vi "conditionalCheck.vi"(10 "State in":T1, 11 "CheckData in in":refnum<class "CheckData.lvclass">[](array[class])) -> (3 "CheckData out":refnum<class "CheckData.lvclass">[](array[class]))   [LabVIEW 2018, in "CheckData.lvclass"]
uses:
  CheckData.lvclass
  TypeDef_ControlState.ctl
  CheckData.lvclass/CheckData.ctl
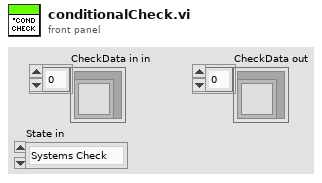
[diagram p1: front panel]
types:
  T1 = typedef "TypeDef_ControlState.ctl" = enum16{"Systems Check", "Idle", "Ready", "Pushing", "Coast", "Braking", "Fault", "Shutdown", "Service", "Precharge", "Blank"}
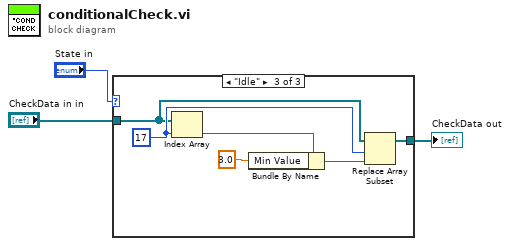
[diagram p0: block diagram]
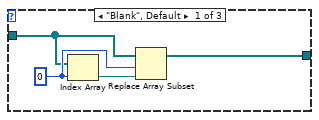
[diagram p2: hidden frame]
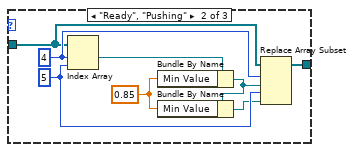
[diagram p3: hidden frame]
diagram:
  n1 = case shown="\"Idle\"" "State in" {
    tunnel: "CheckData in in" -> [w5 w14 w20]
    tunnel: [w4 w13 w19] -> w1
    frame "Blank", Default {
      w6 = 0 ("index")
      n2 = Index Array(array=w5, index=w6) -> (element=w7:refnum<class "CheckData.lvclass">)
      n3 = Replace Array Subset(array=w5, new element=w7, index=w6) -> (w4:refnum<class "CheckData.lvclass">[])
    }
    frame "Ready", "Pushing" {
      w11 = 5 ("index")
      w8 = 0.85 ("Min Value")
      w15 = 4 ("index")
      n4 = Index Array(array=w14, index #1=w15, index #2=w11) -> (element #1=w12:refnum<class "CheckData.lvclass">)  [unwired: 1 out]
      n5 = Bundle By Name(cluster=w12, "Min Value"=w8) -> (w10:refnum<class "CheckData.lvclass">)
      n6 = Bundle By Name(cluster=w10, "Min Value"=w8) -> (w9:refnum<class "CheckData.lvclass">)
      n7 = Replace Array Subset(array=w14, new element #1=w10, index #1=w15, new element #2=w9, index #2=w11) -> (w13:refnum<class "CheckData.lvclass">[])
    }
    frame "Idle" {
      w21 = 17 ("index")
      n8 = Index Array(array=w20, index=w21) -> (element=w18:refnum<class "CheckData.lvclass">)
      n9 = Bundle By Name(cluster=w18, "Min Value"=3.0) -> (w17:refnum<class "CheckData.lvclass">)
      n10 = Replace Array Subset(array=w20, new element=w17, index=w21) -> (w19:refnum<class "CheckData.lvclass">[])
    }
  }
  "CheckData out" <- w1
